vi "tcsOfc_cancelCallback_logEvent_errorCode.vi"(8 "error in (no error)":errorcluster) -> (0 "error out":errorcluster, 3 "function return":i32)   [LabVIEW 2016, in "SALLV_tcsOfc.lvlib"]
doc: "int tcsOfc_shm_cancelCallback_logevent_errorCodeLV();"
uses:
  SALLV_tcsOfc.lvlib
  SALLV_tcsOfc.so
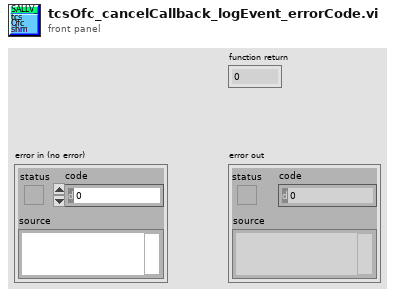
[diagram p1: front panel]
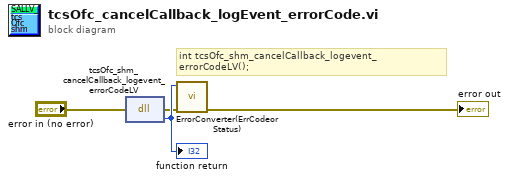
[diagram p0: block diagram]
diagram:
  # "int tcsOfc_shm_cancelCallback_logevent_errorCodeLV();"
  n1 = dll-call lib="home/andres/Desktop/SAL_tcsOfc/SALLV_tcsOfc.*" fn="tcsOfc_shm_cancelCallback_logevent_errorCodeLV"(error in="error in (no error)") -> (error out=w2:errorcluster, w4:i32)  [unwired: 2 in, 1 out]
  "function return" <- w4
  n2 = call "ErrorConverter(ErrCodeorStatus).vi"("error in (no error)"=w2, "error code"=w4) -> ("error out"=→"error out":errorcluster)  [unwired: 9 in]
